vi "Untitled 3.vi"() -> ()   [LabVIEW 2020]
panel:
  in  "DUR":bool
  out "Kırmızı (Araç)":bool
  out "Sarı (Araç)":bool
  out "Yeşil (Araç)":bool
  out "Kırmızı (yaya)":bool
  out "Yeşil (yaya)":bool
  in  "PROGRAMI\n DURDUR":bool
  # "Ahmed Göktuğ Aydın - 200208054"
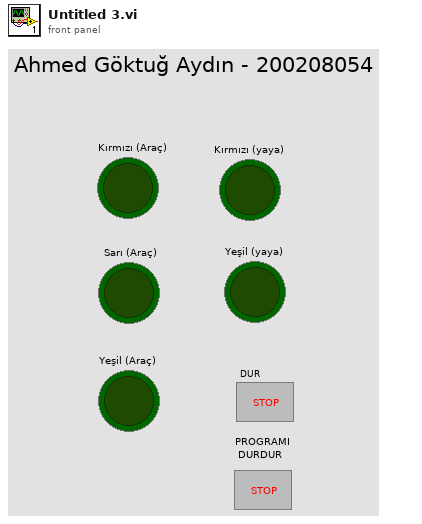
[diagram p1: front panel]
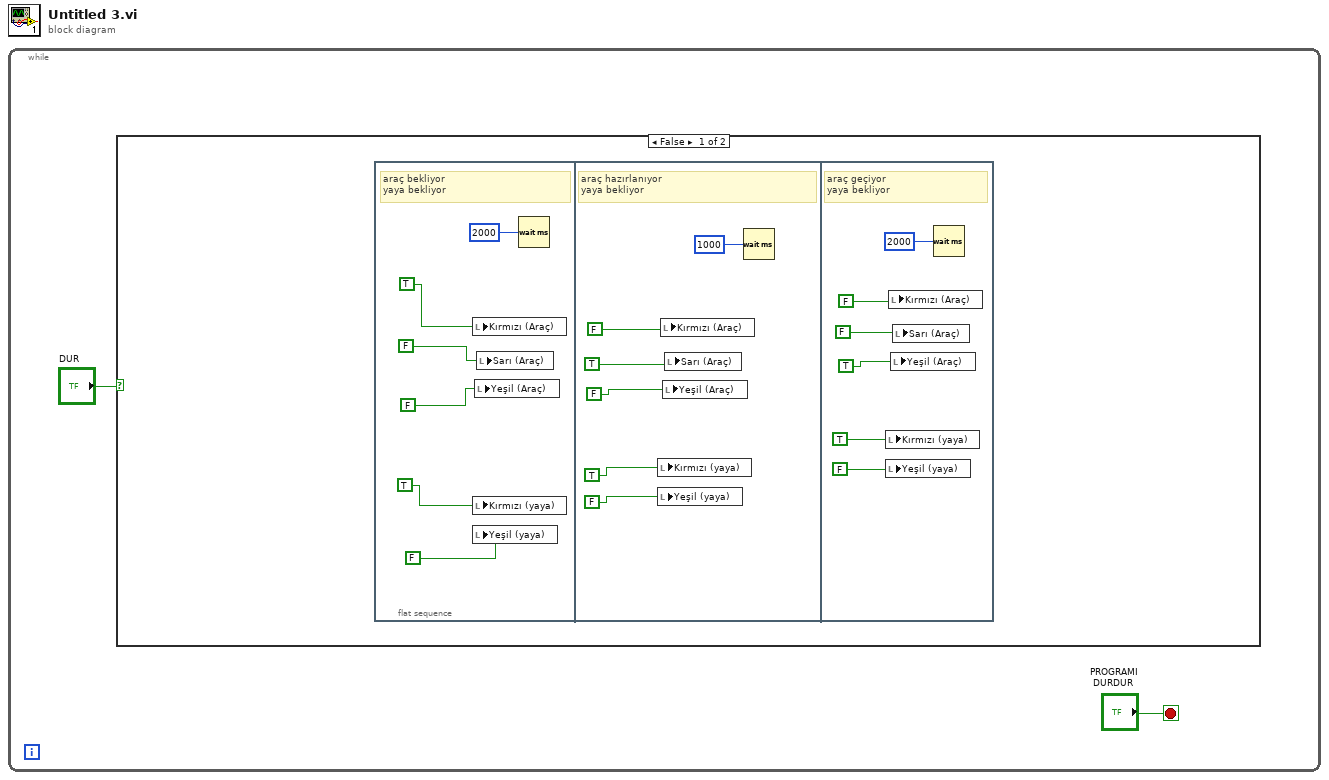
[diagram p0: block diagram]
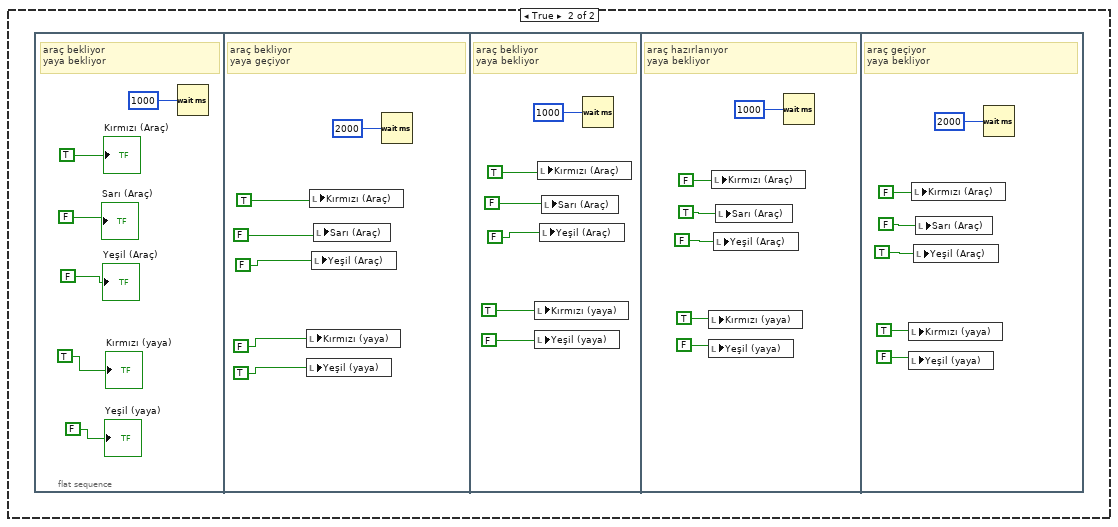
[diagram p2: hidden frame]
diagram:
  n1 = while {
    stop <- "PROGRAMI\n DURDUR" stop-if-true
    n2 = case shown="False" "DUR" {
      frame False {
        n3 = flat-sequence {
          frame #0 {
            # "araç bekliyor\nyaya bekliyor"
            n4 = local write "Kırmızı (Araç)"(TRUE) -> ()
            n5 = local write "Kırmızı (yaya)"(TRUE) -> ()
            n6 = local write "Yeşil (yaya)"(FALSE) -> ()
            n7 = local write "Yeşil (Araç)"(FALSE) -> ()
            n8 = local write "Sarı (Araç)"(FALSE) -> ()
            n9 = Wait (ms)(milliseconds to wait=2000) -> ()  [unwired: 1 out]
          }
          frame #1 {
            # "araç hazırlanıyor \nyaya bekliyor"
            n10 = local write "Kırmızı (yaya)"(TRUE) -> ()
            n11 = local write "Yeşil (yaya)"(FALSE) -> ()
            n12 = local write "Kırmızı (Araç)"(FALSE) -> ()
            n13 = local write "Yeşil (Araç)"(FALSE) -> ()
            n14 = local write "Sarı (Araç)"(TRUE) -> ()
            n15 = Wait (ms)(milliseconds to wait=1000) -> ()  [unwired: 1 out]
          }
          frame #2 {
            # "araç geçiyor\nyaya bekliyor"
            n16 = local write "Kırmızı (yaya)"(TRUE) -> ()
            n17 = local write "Yeşil (yaya)"(FALSE) -> ()
            n18 = local write "Kırmızı (Araç)"(FALSE) -> ()
            n19 = local write "Yeşil (Araç)"(TRUE) -> ()
            n20 = local write "Sarı (Araç)"(FALSE) -> ()
            n21 = Wait (ms)(milliseconds to wait=2000) -> ()  [unwired: 1 out]
          }
        }
      }
      frame True {
        n22 = flat-sequence {
          frame #0 {
            # "araç bekliyor\nyaya bekliyor"
            n23 = Wait (ms)(milliseconds to wait=1000) -> ()  [unwired: 1 out]
            "Kırmızı (Araç)" <- TRUE
            "Sarı (Araç)" <- FALSE
            "Yeşil (Araç)" <- FALSE
            "Kırmızı (yaya)" <- TRUE
            "Yeşil (yaya)" <- FALSE
          }
          frame #1 {
            # "araç bekliyor\nyaya geçiyor"
            n24 = local write "Kırmızı (yaya)"(FALSE) -> ()
            n25 = local write "Yeşil (yaya)"(TRUE) -> ()
            n26 = local write "Kırmızı (Araç)"(TRUE) -> ()
            n27 = local write "Yeşil (Araç)"(FALSE) -> ()
            n28 = local write "Sarı (Araç)"(FALSE) -> ()
            n29 = Wait (ms)(milliseconds to wait=2000) -> ()  [unwired: 1 out]
          }
          frame #2 {
            # "araç bekliyor\nyaya bekliyor"
            n30 = local write "Kırmızı (yaya)"(TRUE) -> ()
            n31 = local write "Yeşil (yaya)"(FALSE) -> ()
            n32 = local write "Kırmızı (Araç)"(TRUE) -> ()
            n33 = local write "Yeşil (Araç)"(FALSE) -> ()
            n34 = local write "Sarı (Araç)"(FALSE) -> ()
            n35 = Wait (ms)(milliseconds to wait=1000) -> ()  [unwired: 1 out]
          }
          frame #3 {
            # "araç hazırlanıyor\nyaya bekliyor"
            n36 = local write "Kırmızı (yaya)"(TRUE) -> ()
            n37 = local write "Yeşil (yaya)"(FALSE) -> ()
            n38 = local write "Kırmızı (Araç)"(FALSE) -> ()
            n39 = local write "Yeşil (Araç)"(FALSE) -> ()
            n40 = local write "Sarı (Araç)"(TRUE) -> ()
            n41 = Wait (ms)(milliseconds to wait=1000) -> ()  [unwired: 1 out]
          }
          frame #4 {
            # "araç geçiyor\nyaya bekliyor"
            n42 = local write "Kırmızı (yaya)"(TRUE) -> ()
            n43 = local write "Yeşil (yaya)"(FALSE) -> ()
            n44 = local write "Kırmızı (Araç)"(FALSE) -> ()
            n45 = local write "Yeşil (Araç)"(TRUE) -> ()
            n46 = local write "Sarı (Araç)"(FALSE) -> ()
            n47 = Wait (ms)(milliseconds to wait=2000) -> ()  [unwired: 1 out]
          }
        }
      }
    }
  }
